vi "PID17.vi"() -> ()   [LabVIEW 2011]
uses:
  <vilib>/DAQmx/read.llb/DAQmx Read (Analog 1D DBL 1Chan NSamp).vi
  <vilib>/DAQmx/write.llb/DAQmx Write (Analog DBL 1Chan 1Samp).vi
  <vilib>/DAQmx/create/channels.llb/DAQmx Create Channel (AI-Voltage-Basic).vi
  <vilib>/DAQmx/configure/timing.llb/DAQmx Timing (Sample Clock).vi
  <vilib>/DAQmx/create/channels.llb/DAQmx Create Channel (AO-Voltage-Basic).vi
  <vilib>/DAQmx/miscellaneous.llb/DAQmx Fill In Error Info.vi
  <vilib>/express/express arith-compare/Formula/XNode/ExpressFormulaBlockNode.xnode
  <vilib>/Analysis/NI_AALBase.lvlib
  Program Files (x86)/National Instruments/LabVIEW 2011/resource/objmgr/daqmx.rc
panel:
  in  "error in":cluster{"status":bool}
  in  "?":T1(tab)
  out "Time":dbl
  out "Thermistor Back":dbl
  out "Thermistor Block":dbl
  out "Vial Ramp rate":dbl format="%#_3g"
  in  "stop":bool
  out "XY Graph":cluster{"Y":dbl[], "Y":dbl[]}[](graph)
  out "Setpoint":dbl
  in  "Zero":dbl=-0.6
  in  "Pole":dbl=-10000000000000.0
  in  "PID Heating":T2={"proportional gain (Kc)"=25.0, "integral time (Ti, s)"=6.0, "derivative time (Td, s)"=0.0} {"derivative time (Td, s)" format="%.3f"; "integral time (Ti, s)" format="%.3f"; "proportional gain (Kc)" format="%.3f"}
  out "Set Pt RampRate":dbl
  out "Error":dbl
  in  "PID Cooling":T2={"proportional gain (Kc)"=25.0, "integral time (Ti, s)"=6.0, "derivative time (Td, s)"=0.0} {"derivative time (Td, s)" format="%.3f"; "integral time (Ti, s)" format="%.3f"; "proportional gain (Kc)" format="%.3f"}
  out "Controller output":cluster{"Time Out":dbl[], dbl[]}(graph)
  out "Power Circuit":cluster{"Time Out":dbl[], dbl[]}(graph)
  out "Voltage":dbl
  out "Ave RR Up":dbl
  out "Ave RR Down":dbl
  in  "A 9":dbl=54.0
  in  "T 15":dbl=5.0
  in  "T 14":dbl=5.0
  in  "A 8":dbl=90.0
  in  "A 7":dbl=96.5
  in  "A 6":dbl=99.0
  in  "A 5":dbl=75.0
  in  "A 4":dbl=69.5
  in  "A 3":dbl=69.0
  in  "A 2":dbl=60.0
  in  "A 1":dbl=57.5
  in  "Aa 6":dbl=54.0
  in  "Aa 5":dbl=85.0
  in  "Aa 4":dbl=96.5
  in  "Aa 3":dbl=99.0
  in  "Aa 2":dbl=80.0
  in  "Aa 1":dbl=51.5
  in  "T 13":dbl=5.0
  in  "T 12":dbl=5.0
  in  "T 11":dbl=20.0
  in  "T 10":dbl=5.0
  in  "T 9":dbl=5.0
  in  "T 8":dbl=5.0
  in  "T 7":dbl=5.0
  in  "T 6":dbl=20.0
  in  "T 5":dbl=5.0
  in  "T 4":dbl=5.0
  in  "T 3":dbl=20.0
  in  "T 2":dbl=5.0
  in  "T 1":dbl=30.0
  in  "Ta 10":dbl=5.0
  in  "Ta 9":dbl=15.0
  in  "Ta 8":dbl=13.0
  in  "Ta 7":dbl=2.0
  in  "Ta 6":dbl=25.0
  in  "Ta 5":dbl=5.0
  in  "Ta 4":dbl=10.0
  in  "Ta 3":dbl=10.0
  in  "Ta 2":dbl=2.0
  in  "Ta 1":dbl=30.0
  in  "Graph Range":dbl=150.0
  out "Rate":dbl
  in  "Period(ms)":dbl=20.0
  out "time":dbl
  # "PID"
  # "Lead-Lag Compensator"
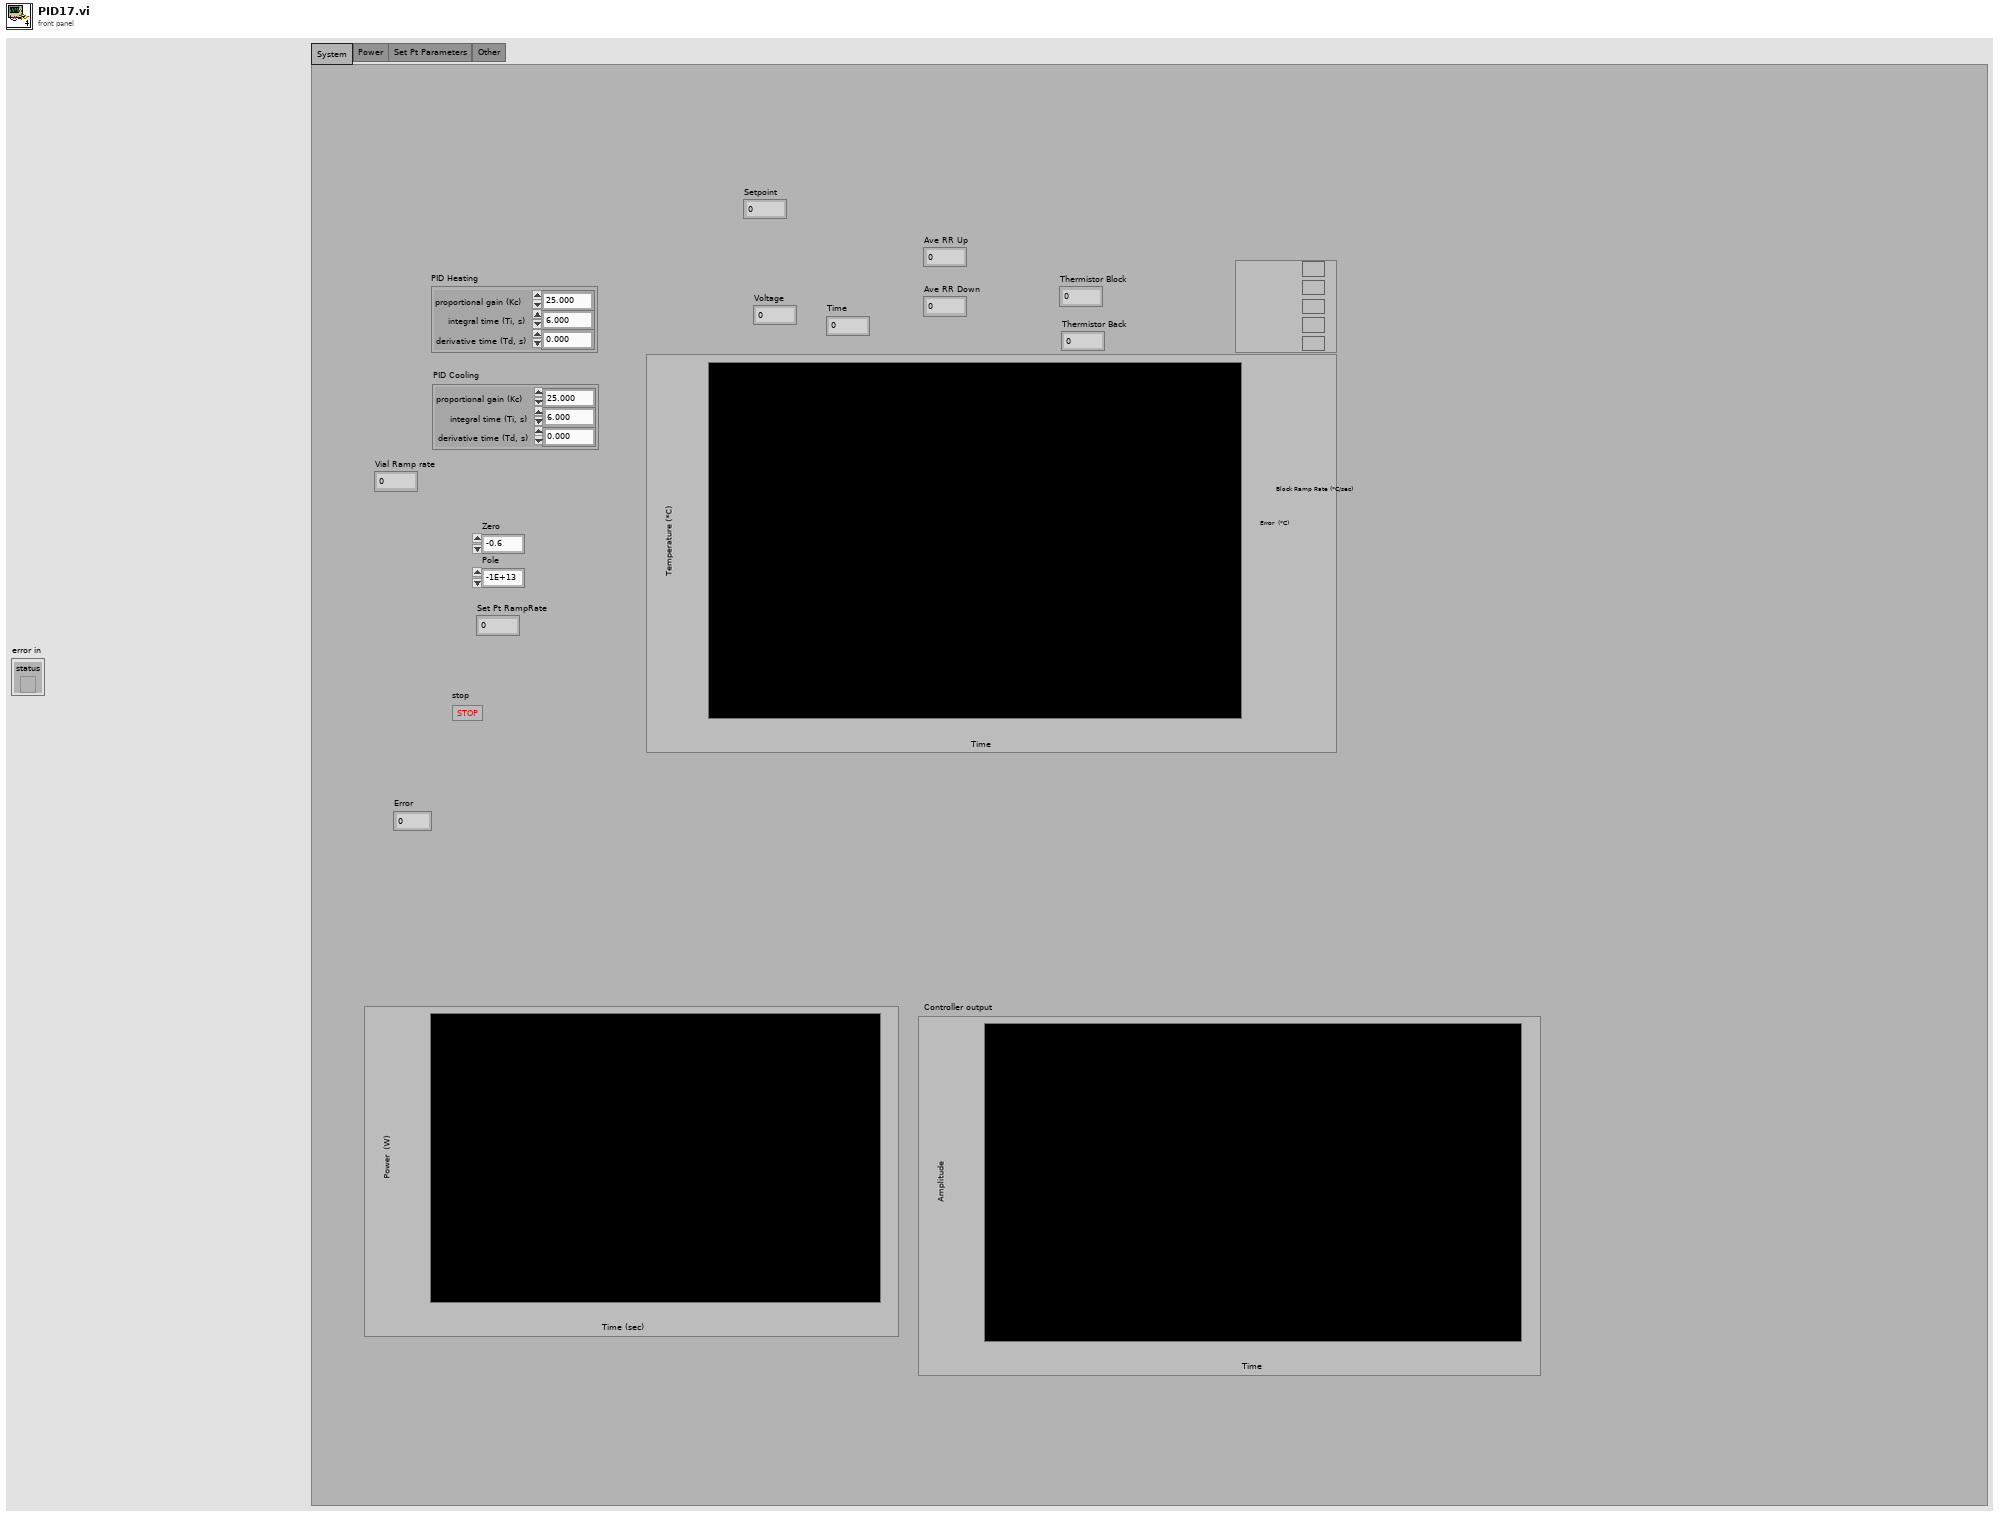
[diagram p1: front panel]
types:
  T1 = enum32{"System", "Power", "Set Pt Parameters", "Other"}
  T2 = cluster{"proportional gain (Kc)":dbl, "integral time (Ti, s)":dbl, "derivative time (Td, s)":dbl}
  T3 = enum16{"open", "replace", "create", "open or create", "replace or create", "replace or create with confirmation"}
  T4 = cluster{"x":dbl, "T1":dbl, "T2":dbl, "T3":dbl, "T4":dbl, "Te1":dbl, "Te2":dbl, "Te3":dbl, "Te4":dbl}
  T5 = cluster{"Ta 1":dbl, "Ta 2":dbl, "Ta 3":dbl, "Ta 4":dbl, "Ta 5":dbl, "Ta 6":dbl, "Ta 7":dbl, "Ta 8":dbl, "Ta 9":dbl, "Ta 10":dbl}
  T6 = cluster{"T 1":dbl, "T 2":dbl, "T 3":dbl, "T 4":dbl, "T 5":dbl, "T 6":dbl, "T 7":dbl, "T 8":dbl, "T 9":dbl, "T 10":dbl, "T 11":dbl, "T 12":dbl, "T 13":dbl, "T 14":dbl, "T 15":dbl}
  T7 = cluster{"Aa 1":dbl, "Aa 2":dbl, "Aa 3":dbl, "Aa 4":dbl, "Aa 5":dbl, "Aa 6":dbl, "A 1":dbl, "A 2":dbl, "A 3":dbl, "A 4":dbl, "A 5":dbl, "A 6":dbl, "A 7":dbl, "A 8":dbl, "A 9":dbl}
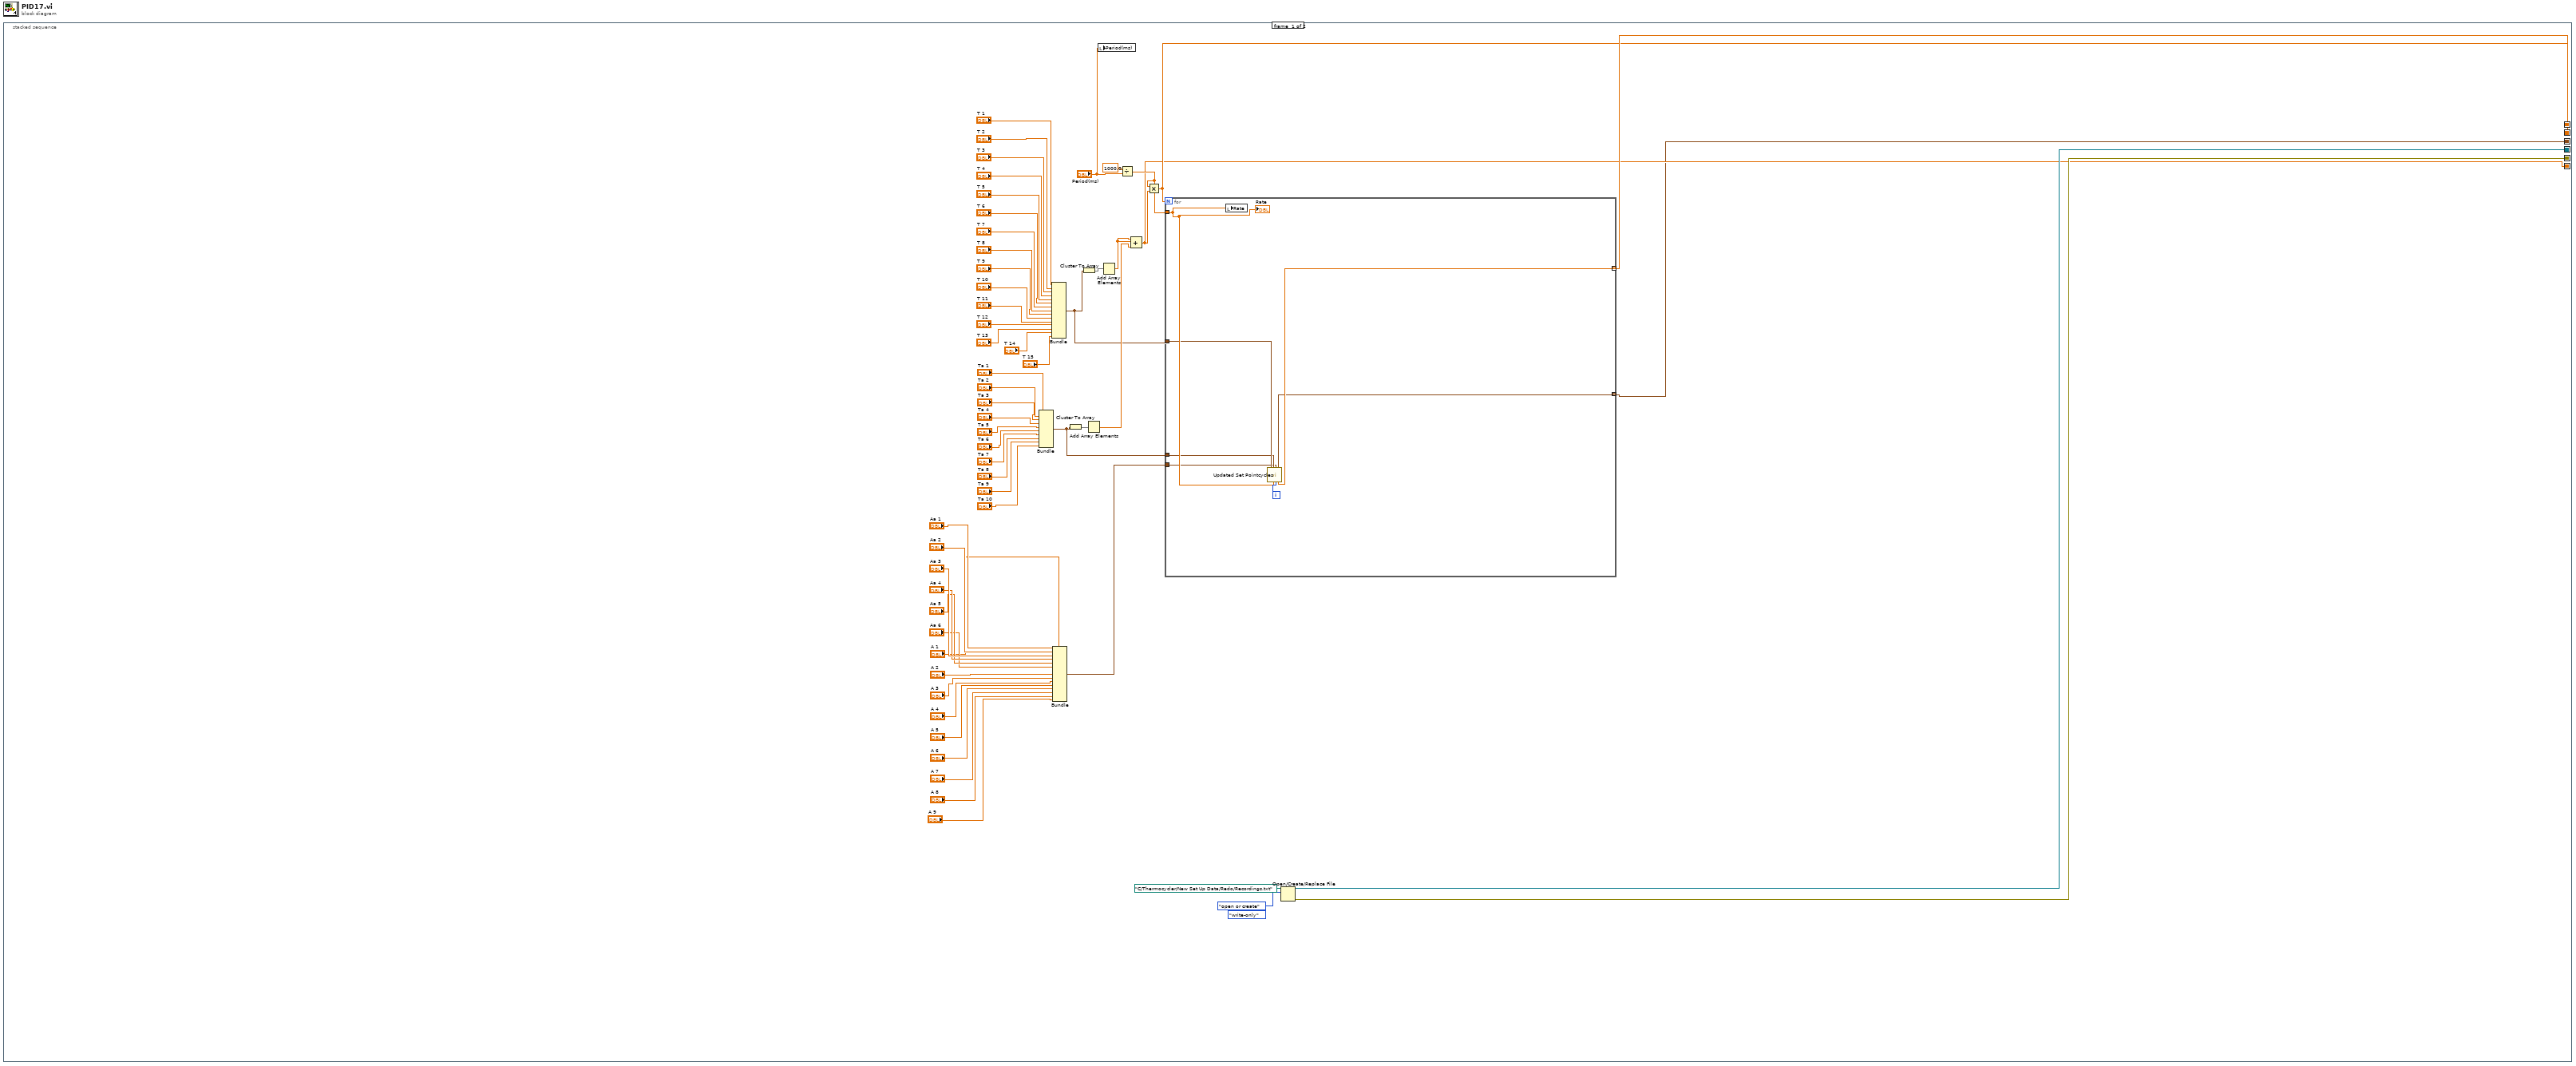
[diagram p0: block diagram]
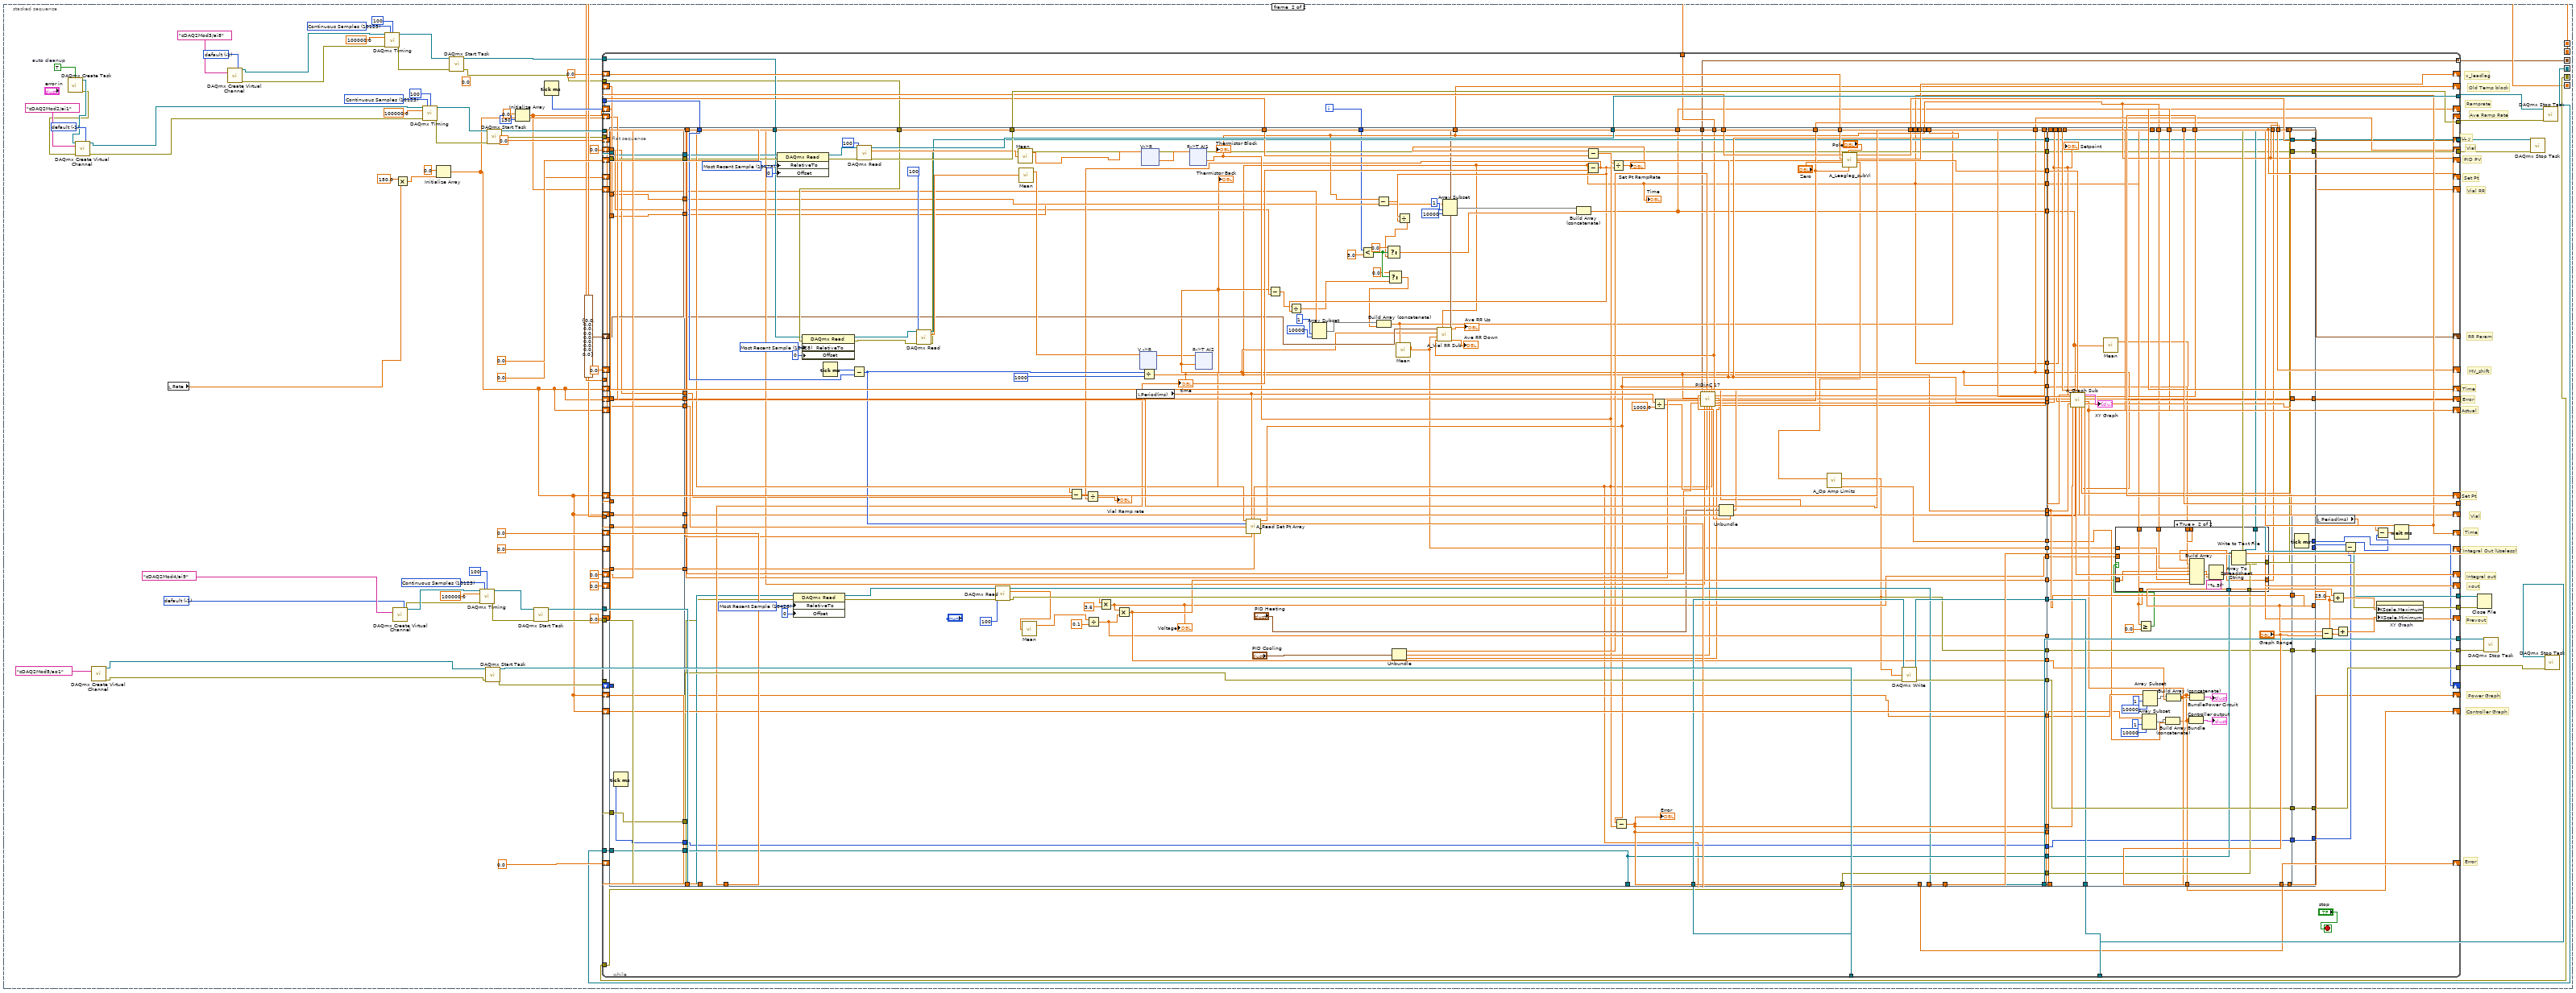
[diagram p2: hidden frame]
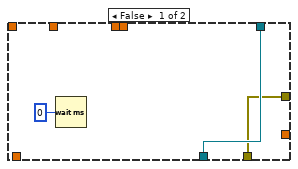
[diagram p3: hidden frame]
diagram:
  n1 = stacked-sequence {
    seq-local: [w57 _] -> [_ w132]
    seq-local: [w54 _] -> [_ w130]
    seq-local: [w4 _] -> [_ w66]
    seq-local: [w52 _] -> [_ w120]
    seq-local: [w51 _] -> [_ w119]
    seq-local: [w49 _] -> [_ w87]
    frame #0 {
      (unwired) enum16{"read/write", "read-only", "write-only"}."write-only" ("access (0:read/write)")
      n2 = Bundle("Ta 1"="Ta 1", "Ta 2"="Ta 2", "Ta 3"="Ta 3", "Ta 4"="Ta 4", "Ta 5"="Ta 5", "Ta 6"="Ta 6", "Ta 7"="Ta 7", "Ta 8"="Ta 8", "Ta 9"="Ta 9", "Ta 10"="Ta 10") -> (w20:T5)  [unwired: 1 in]
      n3 = Bundle("T 1"="T 1", "T 2"="T 2", "T 3"="T 3", "T 4"="T 4", "T 5"="T 5", "T 6"="T 6", "T 7"="T 7", "T 8"="T 8", "T 9"="T 9", "T 10"="T 10", "T 11"="T 11", "T 12"="T 12", "T 13"="T 13", "T 14"="T 14", "T 15"="T 15") -> (w21:T6)  [unwired: 1 in]
      n4 = Bundle("Aa 1"="Aa 1", "Aa 2"="Aa 2", "Aa 3"="Aa 3", "Aa 4"="Aa 4", "Aa 5"="Aa 5", "Aa 6"="Aa 6", "A 1"="A 1", "A 2"="A 2", "A 3"="A 3", "A 4"="A 4", "A 5"="A 5", "A 6"="A 6", "A 7"="A 7", "A 8"="A 8", "A 9"="A 9") -> (w5:T7)  [unwired: 1 in]
      n5 = Cluster To Array(cluster=w20) -> (array=w23:dbl[])
      n6 = Cluster To Array(cluster=w21) -> (array=w35:dbl[])
      n7 = Add Array Elements(numeric array=w23) -> (sum=w22:dbl)
      n8 = local write "Period(ms)"("Period(ms)") -> ()
      n9 = Add Array Elements(numeric array=w35) -> (sum=w34:dbl)
      n10 = Divide(x=1000.0, y="Period(ms)") -> (x/y=w55:dbl)
      n11 = Compound Arithmetic op=ADD(w34, w34, w22) -> (w49:dbl)
      n12 = Multiply(x=w55, y=w49) -> (x*y=w54:dbl)
      n13 = for {
        N: w54 -> [_]
        tunnel: w55 -> [w63]
        tunnel: [w65] -> w57 mode=indexing
        tunnel: w21 -> [w62]
        tunnel: w20 -> [w61]
        tunnel: w5 -> [w60]
        tunnel: [w59] -> w4 mode=indexing
        i -> [w64]
        n14 = local write "Rate"(w63) -> ()
        n15 = call "Updated Set Pointcycles.vi"("Time2"=w62, "Time1"=w61, "rate"=w63, "Amp"=w60, "i"=w64) -> ("Gain times"=w59:cluster{dbl, dbl, dbl, dbl, dbl, dbl}, "y"=w65:dbl)  [unwired: 13 in]
        "Rate" <- w63
      }
      n16 = Open/Create/Replace File(file path (use dialog)=path "C:/Thermocycler/New Set Up Data/Redo/Recordings.txt", operation (0:open)=T3."open or create") -> (refnum out=w52:refnum<file>, error out=w51:errorcluster)  [unwired: 2 in, 3 out]
    }
    frame #1 {
      w81 = -1 items=["default"=-1, "RSE"=10083, "NRSE"=10078, "Differential"=10106, "Pseudodifferential"=12529] ("input terminal configuration")
      (unwired) 0.0 ("y")
      w84 = 10123 items=["Finite Samples"=10178, "Continuous Samples"=10123, "Hardware Timed Single Point"=12522] ("sample mode")
      w103 = TRUE  # auto cleanup
      w105 = -1 items=["default"=-1, "RSE"=10083, "NRSE"=10078, "Differential"=10106, "Pseudodifferential"=12529] ("input terminal configuration")
      w112 = 10123 items=["Finite Samples"=10178, "Continuous Samples"=10123, "Hardware Timed Single Point"=12522] ("sample mode")
      w115 = -1 items=["default"=-1, "RSE"=10083, "NRSE"=10078, "Differential"=10106, "Pseudodifferential"=12529] ("input terminal configuration")
      w141 = 10123 items=["Finite Samples"=10178, "Continuous Samples"=10123, "Hardware Timed Single Point"=12522] ("sample mode")
      # "Vial RR"
      # "Vial"
      # "RR Param"
      # "Ave Ramp Rate"
      # "Ramprate"
      # "Old Temp block"
      # "Controller Graph"
      # "Power Graph"
      # "MV_shift"
      # "Prevout"
      # "xout"
      # "Integral out"
      # "Vial"
      # "Time"
      # "Integral Out (Useless)"
      # "Error"
      # "PID PV"
      # "Set Pt"
      # "x_leadlag"
      # "Set Pt"
      # "Actual"
      # "Error"
      # "Time"
      # "LL y"
      n17 = call <vilib>:"DAQmx Create Task.vi"("auto cleanup"=w103) -> ("task out"=w102:refnum<k21>, "error out"=w101:errorcluster)  [unwired: 13 in]
      n18 = call-poly <vilib>:"DAQmx Create Virtual Channel.vi"("task in"=w102, "input terminal configuration"=w105, "physical channels"=tag "cDAQ2Mod2/ai1", "error in"=w101) -> ("task out"=w86:refnum<k21>, "error out"=w85:errorcluster)  [unwired: 10 in]
      n19 = call-poly <vilib>:"DAQmx Create Virtual Channel.vi"("physical channels"=tag "cDAQ2Mod5/ao1") -> ("task out"=w95:refnum<k21>, "error out"=w94:errorcluster)  [unwired: 13 in]
      n20 = local read "Rate"() -> (w125:dbl)
      n21 = call-poly <vilib>:"DAQmx Create Virtual Channel.vi"("input terminal configuration"=w81, "physical channels"=tag "cDAQ2Mod3/ai8") -> ("task out"=w77:refnum<k21>, "error out"=w76:errorcluster)  [unwired: 12 in]
      n22 = call-poly <vilib>:"DAQmx Timing.vi"("task/channels in"=w77, "sample mode"=w84, "samples per channel"=100, "rate"=100000.0, "error in"=w76) -> ("task out"=w79:refnum<k21>, "error out"=w78:errorcluster)  [unwired: 9 in]
      n23 = call-poly <vilib>:"DAQmx Create Virtual Channel.vi"("input terminal configuration"=w115, "physical channels"=tag "cDAQ2Mod4/ai9") -> ("task out"=w114:refnum<k21>, "error out"=w113:errorcluster)  [unwired: 12 in]
      n24 = Multiply(x=150.0, y=w125) -> (x*y=w124:dbl)
      n25 = call-poly <vilib>:"DAQmx Timing.vi"("task/channels in"=w86, "sample mode"=w141, "samples per channel"=100, "rate"=100000.0, "error in"=w85) -> ("task out"=w99:refnum<k21>, "error out"=w98:errorcluster)  [unwired: 9 in]
      n26 = Initialize Array(0.0 ("element"), w124) -> (w69:dbl[])
      n27 = call <vilib>:"DAQmx Start Task.vi"("task/channels in"=w79, "error in"=w78) -> ("task out"=w75:refnum<k21>, "error out"=w74:errorcluster)  [unwired: 12 in]
      n28 = call-poly <vilib>:"DAQmx Timing.vi"("task/channels in"=w114, "sample mode"=w112, "samples per channel"=100, "rate"=100000.0, "error in"=w113) -> ("task out"=w97:refnum<k21>, "error out"=w96:errorcluster)  [unwired: 9 in]
      n29 = call <vilib>:"DAQmx Start Task.vi"("task/channels in"=w95, "error in"=w94) -> ("task out"=w131:refnum<k21>, "error out"=w137:errorcluster)  [unwired: 12 in]
      n30 = call <vilib>:"DAQmx Start Task.vi"("task/channels in"=w99, "error in"=w98) -> ("task out"=w139:refnum<k21>, "error out"=w100:errorcluster)  [unwired: 12 in]
      n31 = Initialize Array(0.0 ("element"), 150 ("dimension size")) -> (w68:dbl[])
      n32 = call <vilib>:"DAQmx Start Task.vi"("task/channels in"=w97, "error in"=w96) -> ("task out"=w109:refnum<k21>, "error out"=w108:errorcluster)  [unwired: 12 in]
      n33 = Tick Count (ms)() -> (millisecond timer value=w144:u32)
      n34 = while {
        tunnel: w144 -> [w280]
        shift-right: [w193] -> _
        shift-left: 0.0 ("data") -> [w258]
        shift-right: [w225] -> _
        shift-left: 0.0 -> [w277]
        tunnel: w100 -> [w275]
        tunnel: w139 -> [w274]
        tunnel: w137 -> [w271]
        tunnel: [w269] -> w136
        tunnel: [w266] -> w135
        tunnel: [w265] -> w134
        tunnel: [w264] -> w133
        tunnel: w132 -> [w263]
        tunnel: w131 -> [w261]
        tunnel: w130 -> [w259]
        shift-right: [w224] -> _
        shift-left: 0.0 ("Setpoint") -> [w233]
        shift-right: [w248] -> _
        shift-left: 0.0 ("Integral") -> [w255]
        tunnel: [w254] -> _
        shift-right: [w253] -> _
        shift-left: 0.0 -> [w252]
        shift-right: [w226] -> _
        shift-left: 0.0 ("y") -> [w250]
        shift-right: [w230] -> _
        shift-left: w69 -> [w246]
        shift-right: [w229] -> _
        shift-left: w69 -> [w243]
        shift-right: [w227] -> _
        shift-left: w69 -> [w242]
        shift-right: [w228] -> _
        shift-left: w69 -> [w247]
        shift-right: [w236] -> _
        shift-left: 0.0 ("LL x out") -> [w235]
        tunnel: w120 -> [w223]
        tunnel: w119 -> [w220]
        tunnel: [w218] -> w118
        tunnel: [w217] -> w117
        tunnel: w109 -> [w216]
        tunnel: w108 -> [w215]
        tunnel: [w214] -> w107
        tunnel: [w213] -> w106
        shift-right: [w208] -> _
        shift-left: w69 -> [w207]
        shift-right: [w203] -> _
        shift-left: 0.0 ("Integral out") -> [w199]
        shift-right: [w202] -> _
        shift-left: 0.0 ("x out") -> [w198]
        shift-right: [w201] -> _
        shift-left: 0.0 ("prev out") -> [w200]
        shift-right: [w197] -> _
        shift-left: 0.0 ("MV") -> [w196]
        shift-right: [w195] -> _
        shift-left: 0.0 ("Result") -> [w151]
        shift-right: [w187] -> _
        shift-left: _ -> [w186]
        shift-right: [w180] -> _
        shift-left: w69 -> [w182]
        shift-right: [w178] -> _
        shift-left: w69 -> [w179]
        tunnel: w87 -> [w175]
        tunnel: w75 -> [w174]
        tunnel: w74 -> [w167]
        tunnel: [w171] -> w73
        tunnel: [w168] -> w72
        shift-right: [w166] -> _
        shift-left: _ -> [w165]
        shift-right: [w163] -> _
        shift-left: w68 -> [w162]
        shift-right: [w159] -> _
        shift-left: w69 -> [w157]
        shift-right: [w153] -> _
        shift-left: T4 {"x"=0.0, "T1"=0.0, "T2"=0.0, "T3"=0.0, "T4"=0.0, "Te1"=0.0, "Te2"=0.0, "Te3"=0.0, "Te4"=0.0} ("Param out") -> [w152]
        shift-right: [w150] -> _
        shift-left: w68 -> [w149]
        tunnel: w66 -> [w145] mode=indexing
        i -> [w147]
        stop <- "stop" stop-if-true
        w241 = 25.0 ("y")
        n35 = flat-sequence {
          tunnel: [w293] -> w276
          tunnel: w275 -> [w293]
          tunnel: w274 -> [w290]
          tunnel: [w290] -> w273
          tunnel: [w292] -> w272
          tunnel: w271 -> [w292]
          tunnel: w263 -> [w291]
          tunnel: [w291] -> w262
          tunnel: [w289] -> w260
          tunnel: w259 -> [w289]
          tunnel: [w288] -> w256
          tunnel: w255 -> [w288]
          tunnel: w223 -> [w287]
          tunnel: [w287] -> w222
          tunnel: w207 -> [w286]
          tunnel: [w286] -> w206
          tunnel: [w285] -> w194
          tunnel: w151 -> [w285]
          tunnel: [w284] -> w191
          tunnel: w186 -> [_]
          tunnel: w165 -> [w283]
          tunnel: [w283] -> w164
          tunnel: w162 -> [w282]
          tunnel: [w282] -> w161
          tunnel: w157 -> [w281]
          tunnel: [w281] -> w156
          tunnel: w280 -> [w414]
          tunnel: [w348] -> w279
          tunnel: [w296] -> w278
          tunnel: [w296] -> w225
          tunnel: w277 -> [w391]
          tunnel: w276 -> [w386]
          tunnel: w273 -> [w412]
          tunnel: w272 -> [w411]
          tunnel: [w410] -> w270
          tunnel: [w409] -> w267
          tunnel: [w408] -> w265
          tunnel: [w407] -> w264
          tunnel: w262 -> [w406]
          tunnel: w261 -> [w405]
          tunnel: w260 -> [w404]
          tunnel: [w331] -> w193
          tunnel: w258 -> [w403]
          tunnel: [w331] -> w257
          tunnel: w233 -> [w395]
          tunnel: [w348] -> w224
          tunnel: [w402] -> w248
          tunnel: w256 -> [w401]
          tunnel: [w331] -> _
          tunnel: [w394] -> w253
          tunnel: w252 -> [_]
          tunnel: [w394] -> w251
          tunnel: [w397] -> w226
          tunnel: w250 -> [w398]
          tunnel: [w392] -> w236
          tunnel: [w296] -> w245
          tunnel: [w394] -> w244
          tunnel: w235 -> [w393]
          tunnel: w222 -> [w390]
          tunnel: [w390] -> _
          tunnel: [w390] -> w221
          tunnel: w220 -> [w389]
          tunnel: [w389] -> w219
          tunnel: w216 -> [w388]
          tunnel: w215 -> [w385]
          tunnel: [w381] -> w214
          tunnel: [w380] -> w212
          tunnel: [w377] -> w210
          tunnel: [w377] -> w209
          tunnel: w206 -> [w376]
          tunnel: [w376] -> w205
          tunnel: [w308] -> w204
          tunnel: [w370] -> w203
          tunnel: [w369] -> w202
          tunnel: [w368] -> w201
          tunnel: w200 -> [w367]
          tunnel: w199 -> [w366]
          tunnel: w198 -> [w365]
          tunnel: [w364] -> w197
          tunnel: w196 -> [_]
          tunnel: [w308] -> w195
          tunnel: w194 -> [w363]
          tunnel: [w308] -> w192
          tunnel: w191 -> [w358]
          tunnel: [w358] -> w190
          tunnel: w182 -> [w357]
          tunnel: [w357] -> w181
          tunnel: [w355] -> w177
          tunnel: [w354] -> w176
          tunnel: w175 -> [w316]
          tunnel: w174 -> [w335]
          tunnel: [w340] -> w173
          tunnel: [w339] -> w170
          tunnel: w167 -> [w336]
          tunnel: [w331] -> w166
          tunnel: w164 -> [w330]
          tunnel: [w326] -> w163
          tunnel: w161 -> [w327]
          tunnel: [w326] -> w160
          tunnel: w156 -> [w325]
          tunnel: [w325] -> w155
          tunnel: [w322] -> w154
          tunnel: [w319] -> w153
          tunnel: w152 -> [w318]
          tunnel: w151 -> [w314]
          tunnel: [w310] -> w150
          tunnel: w149 -> [w309]
          tunnel: [w299] -> w148
          tunnel: w147 -> [w305]
          tunnel: [w296] -> w146
          tunnel: w145 -> [w295]
          tunnel: w279 -> [w496]
          tunnel: w278 -> [w486]
          tunnel: w270 -> [w509]
          tunnel: [w509] -> w268
          tunnel: w267 -> [w508]
          tunnel: [w508] -> w266
          tunnel: w257 -> [w498]
          tunnel: [w486] -> _
          tunnel: [w496] -> w254
          tunnel: w251 -> [_]
          tunnel: "Graph Range" -> [_]
          tunnel: [w506] -> w228
          tunnel: w247 -> [w505]
          tunnel: w246 -> [w504]
          tunnel: [w468] -> w230
          tunnel: w245 -> [w497]
          tunnel: w244 -> [w503]
          tunnel: w243 -> [w502]
          tunnel: [w501] -> w229
          tunnel: [w500] -> w227
          tunnel: w242 -> [w499]
          tunnel: [w497] -> w240
          tunnel: w225 -> [w493]
          tunnel: w224 -> [w492]
          tunnel: w193 -> [_]
          tunnel: w221 -> [w491]
          tunnel: w219 -> [w490]
          tunnel: [w489] -> w218
          tunnel: [w488] -> w217
          tunnel: w212 -> [w487]
          tunnel: [w487] -> w211
          tunnel: w210 -> [w473]
          tunnel: w209 -> [w485]
          tunnel: [w484] -> w208
          tunnel: w205 -> [w483]
          tunnel: w204 -> [w482]
          tunnel: w193 -> [w481]
          tunnel: w192 -> [w479]
          tunnel: w190 -> [w480]
          tunnel: [w480] -> w189
          tunnel: w181 -> [w472]
          tunnel: [w471] -> w180
          tunnel: w179 -> [w465]
          tunnel: [w464] -> w178
          tunnel: w177 -> [w463]
          tunnel: w176 -> [_]
          tunnel: w173 -> [w462]
          tunnel: [w462] -> w172
          tunnel: w170 -> [w461]
          tunnel: [w461] -> w169
          tunnel: w160 -> [w458]
          tunnel: [w460] -> w158
          tunnel: w155 -> [w459]
          tunnel: w154 -> [w467]
          tunnel: w148 -> [w456]
          tunnel: w146 -> [w455]
          tunnel: [w530] -> w232
          tunnel: [w534] -> w269
          tunnel: w268 -> [w534]
          tunnel: w240 -> [w533]
          tunnel: [w533] -> w238
          tunnel: [w532] -> w213
          tunnel: w211 -> [w532]
          tunnel: w189 -> [w531]
          tunnel: [w531] -> w188
          tunnel: [w530] -> w187
          tunnel: w172 -> [w529]
          tunnel: [w529] -> w171
          tunnel: w169 -> [w528]
          tunnel: [w528] -> w168
          tunnel: [w527] -> w159
          tunnel: w158 -> [w527]
          frame #0 {
            n36 = Tick Count (ms)() -> (millisecond timer value=w284:u32)
          }
          frame #1 {
            w337 = 10428 items=["First Sample"=10424, "Current Read Position"=10425, "Reference Trigger"=10426, "First Pretrigger Sample"=10427, "Most Recent Sample"=10428] ("RelativeTo")
            w382 = 10428 items=["First Sample"=10424, "Current Read Position"=10425, "Reference Trigger"=10426, "First Pretrigger Sample"=10427, "Most Recent Sample"=10428] ("RelativeTo")
            w419 = 10428 items=["First Sample"=10424, "Current Read Position"=10425, "Reference Trigger"=10426, "First Pretrigger Sample"=10427, "Most Recent Sample"=10428] ("RelativeTo")
            n37 = property class="DAQmx Read"(reference=w412, error in=w386, "RelativeTo"=w419, "Offset"=0) -> (reference out=w417:refnum<k21>, error out=w416:errorcluster)
            n38 = property class="DAQmx Read"(reference=w388, error in=w385, "RelativeTo"=w382, "Offset"=0) -> (reference out=w387:refnum<k21>, error out=w384:errorcluster)
            n39 = property class="DAQmx Read"(reference=w335, error in=w336, "RelativeTo"=w337, "Offset"=0) -> (reference out=w334:refnum<k21>, error out=w333:errorcluster)
            n40 = Tick Count (ms)() -> (millisecond timer value=w420:u32)
            n41 = Subtract(x=w420, y=w414) -> (x-y=w396:u32)
            n42 = call-poly <vilib>:"DAQmx Read.vi"("task/channels in"=w417, "number of samples per channel"=100, "error in"=w416) -> ("task out"=w408:refnum<k21>, "data"=w343:dbl[], "error out"=w407:errorcluster)  [unwired: 10 in]
            n43 = call-poly <vilib>:"DAQmx Read.vi"("task/channels in"=w334, "number of samples per channel"=100, "error in"=w333) -> ("task out"=w340:refnum<k21>, "data"=w341:dbl[], "error out"=w339:errorcluster)  [unwired: 10 in]
            n44 = call-poly <vilib>:"DAQmx Read.vi"("task/channels in"=w387, "number of samples per channel"=100, "error in"=w384) -> ("task out"=w381:refnum<k21>, "data"=w345:dbl[], "error out"=w380:errorcluster)  [unwired: 10 in]
            n45 = call <vilib>:"Mean.vi"("X"=w343) -> ("mean"=w347:dbl)  [unwired: 1 out]
            n46 = call <vilib>:"Mean.vi"("X"=w341) -> ("mean"=w375:dbl)  [unwired: 1 out]
            n47 = call <vilib>:"Mean.vi"("X"=w345) -> ("mean"=w344:dbl)  [unwired: 1 out]
            n48 = Divide(x=w344, y=0.1) -> (x/y=w354:dbl)
            n49 = local read "Period(ms)"() -> (w361:dbl)
            n50 = xnode "V ->R"("V"=w375) -> ("Result"=w307:dbl)  [unwired: 1 in, 1 out]
            n51 = xnode "V->R"("V"=w347) -> ("Result"=w422:dbl)  [unwired: 1 in, 1 out]
            n52 = Divide(x=w396, y=1000) -> (x/y=w296:dbl)
            "time" <- w296
            "Time" <- w296
            n53 = xnode "R->T AI1"("R"=w422) -> ("Result"=w331:dbl)  [unwired: 1 in, 1 out]
            "Thermistor Block" <- w331
            n54 = xnode "R->T AI2"("R"=w307) -> ("Result"=w308:dbl)  [unwired: 1 in, 1 out]
            "Thermistor Back" <- w308
            n55 = Subtract(x=w308, y=w363) -> (x-y=w362:dbl)
            n56 = call "A_Read Set Pt Array.vi"("Previous y"=w403, "Period(ms)"=w361, "Result"=w331, "dt"=w396, "y array"=w406, "arraysize"=w404, "Integral in"=w401) -> ("Set Pt Out"=w348:dbl, "Integral out"=w402:dbl)  [unwired: 7 in]
            n57 = Subtract(x=w308, y=w314) -> (x-y=w313:dbl)
            n58 = Array Subset(array=w309, index=1, length=10000) -> (w315:dbl[])
            n59 = Less?(x=w305, y=5.0) -> (x < y?=w303:bool)
            n60 = Subtract(x=w331, y=w330) -> (x-y=w332:dbl)
            n61 = Unbundle("PID Cooling") -> ("proportional gain (Kc)"=w352:dbl, "integral time (Ti, s)"=w350:dbl, "derivative time (Td, s)"=w351:dbl)
            n62 = Array Subset(array=w327, index=1, length=10000) -> (w328:dbl[])
            n63 = Subtract(x=w348, y=w395) -> (x-y=w413:dbl)
            n64 = Subtract(x=w296, y=w391) -> (x-y=w317:dbl)
            n65 = Divide(x=w362, y=w317) -> (x/y=→"Vial Ramp rate":dbl)
            n66 = Divide(x=w313, y=w317) -> (x/y=w298:dbl)
            n67 = Select(t=0.0, s=w303, f=w298) -> (s? t:f=w297:dbl)
            n68 = Build Array (concatenate)(w315, w297) -> (w310:dbl[])
            n69 = call <vilib>:"Mean.vi"("X"=w310) -> ("mean"=w299:dbl)  [unwired: 1 out]
            n70 = Divide(x=w332, y=w317) -> (x/y=w301:dbl)
            n71 = Select(t=0.0, s=w303, f=w301) -> (s? t:f=w300:dbl)
            n72 = call "A_Vial RR Sub.vi"("t"=w296, "TotalTime"=w316, "Vial Slope"=w299, "Vial Temp"=w308, "Param in"=w318) -> ("Ave RR Down"=→"Ave RR Down":dbl, "Param out"=w319:T4, "Ave RR Up"=→"Ave RR Up":dbl)  [unwired: 4 in]
            n73 = Build Array (concatenate)(w328, w300) -> (w326:dbl[])
            n74 = Divide(x=w413, y=w317) -> (x/y=→"Set Pt RampRate":dbl)
            n75 = Subtract(x=w348, y=w331) -> (x-y=w394:dbl)
            "Error" <- w394
            n76 = Divide(x=w361, y=1000.0) -> (x/y=w360:dbl)
            n77 = Unbundle("PID Heating") -> ("proportional gain (Kc)"=w372:dbl, "integral time (Ti, s)"=w373:dbl, "derivative time (Td, s)"=w374:dbl)
            n78 = call "PIDinC 17.vi"("Gain Schedule"=w295, "D"=w374, "Time"=w296, "Integral in"=w366, "prev in"=w367, "I"=w373, "x in"=w365, "P2"=w352, "dt"=w360, "P"=w372, "I2"=w350, "Set Point"=w348, "PV"=w331, "Total Time"=w316, "D2"=w351) -> ("Integral out"=w370:dbl, "MV"=w364:dbl, "prev out"=w368:dbl, "x out"=w369:dbl)  [unwired: 1 in]
            n79 = call "A_Leaglag_subVi.vi"("LL x"=w364, "Pole"="Pole", "Zero"="Zero", "LL x_prev"=w393, "LL y_prev"=w398) -> ("y*inv_gain"=w323:dbl, "LL x out"=w392:dbl, "LL y"=w397:dbl)  [unwired: 4 in]
            n80 = call "A_Op Amp Limits.vi"("Lead Lag"=w323) -> ("Controller Output"=w322:dbl, "Write DAQmx"=w294:dbl)  [unwired: 9 in]
            n81 = Multiply(x=w294, y=3.6) -> (x*y=w355:dbl)
            "Voltage" <- w355
            n82 = Multiply(x=w355, y=w354) -> (x*y=w377:dbl)
            n83 = call-poly <vilib>:"DAQmx Write.vi"("task/channels in"=w405, "data"=w294, "error in"=w411) -> ("task out"=w409:refnum<k21>, "error out"=w410:errorcluster)  [unwired: 10 in, 1 out]
          }
          frame #2 {
            n84 = call "A_Graph Sub.vi"("Set Point Shift"=w505, "New Set Pt"=w496, "Ramp Rate Shift"=w459, "Time Shift"=w504, "New Time"=w497, "New Error"=w503, "New Ramp Rate"=w458, "Error Shift"=w502, "New Actual"=w498, "Actual Shift"=w499, "New Vial"=w482, "Vial Shift"=w483) -> ("Vial Out"=w484:dbl[], "Actual Out"=w500:dbl[], "Graph Out"=→"XY Graph":cluster{dbl[], dbl[]}[], "Set Pt Out"=w506:dbl[], "Ramp Rate Out"=w460:dbl[], "Time Out"=w468:dbl[], "Error Out"=w501:dbl[])  [unwired: 1 in]
            n85 = call <vilib>:"Mean.vi"("X"=w458) -> ("mean"=w457:dbl)  [unwired: 1 out]
            n86 = Greater Or Equal?(x=w493, y=0.0) -> (x >= y?=w494:bool)
            n87 = case shown="True" w494 {
              tunnel: w493 -> [_ _]
              tunnel: w492 -> [_ w516]
              tunnel: w491 -> [w511 w526]
              tunnel: w490 -> [w510 w525]
              tunnel: [w510 w524] -> w489
              tunnel: [w511 w523] -> w488
              tunnel: w485 -> [_ w519]
              tunnel: w481 -> [_ w518]
              tunnel: w479 -> [_ w517]
              tunnel: w463 -> [_ _]
              tunnel: w457 -> [_ w515]
              tunnel: w456 -> [_ w514]
              tunnel: w455 -> [_ w513]
              frame False {
                n88 = Wait (ms)(milliseconds to wait=u32 0) -> ()  [unwired: 1 out]
              }
              frame True {
                n89 = Build Array(w516, w517, w518, w519, w515, w514, w513) -> (w522:dbl[])
                n90 = Array To Spreadsheet String(array=w522, 3:"%.5f" ("format string")) -> (spreadsheet string=w520:string)  [unwired: 1 out]
                n91 = Write to Text File(file (use dialog)=w526, text=w520, error in=w525) -> (refnum out=w523:refnum<file>, error out=w524:errorcluster)  [unwired: 1 in, 1 out]
              }
            }
            n92 = Array Subset(array=w465, index=1, length=10000) -> (w466:dbl[])
            n93 = Array Subset(array=w472, index=1, length=10000) -> (w470:dbl[])
            n94 = Build Array (concatenate)(w466, w467) -> (w464:dbl[])
            n95 = Build Array (concatenate)(w470, w473) -> (w471:dbl[])
            n96 = Bundle("Time Out"=w468, w464) -> (→"Controller output":cluster{"Time Out":dbl[], dbl[]})  [unwired: 1 in]
            n97 = Bundle("Time Out"=w468, w471) -> (→"Power Circuit":cluster{"Time Out":dbl[], dbl[]})  [unwired: 1 in]
            "Setpoint" <- w496
          }
          frame #3 {
            n98 = Tick Count (ms)() -> (millisecond timer value=w530:u32)
          }
        }
        n99 = local read "Period(ms)"() -> (w185:dbl)
        n100 = Subtract(x=w238, y="Graph Range") -> (x-y=w249:dbl)
        n101 = Add(x=w238, y=w241) -> (x+y=w239:dbl)
        n102 = Add(x=w241, y=w249) -> (x+y=w237:dbl)
        n103 = Subtract(x=w232, y=w188) -> (x-y=w183:u32)
        n104 = Subtract(x=w185, y=w183) -> (x-y=w184:dbl)
        n105 = property on="XY Graph" class="XYGraph (strict)"("XScale.Maximum"=w239, "XScale.Minimum"=w237) -> ()  [unwired: 2 in, 2 out]
        n106 = Wait (ms)(milliseconds to wait=w184) -> ()  [unwired: 1 out]
      }
      n107 = Close File(refnum=w117, error in=w118) -> ()  [unwired: 2 out]
      n108 = call <vilib>:"DAQmx Stop Task.vi"("task/channels in"=w107, "error in"=w106) -> ()  [unwired: 12 in, 2 out]
      n109 = call <vilib>:"DAQmx Stop Task.vi"("task/channels in"=w73, "error in"=w72) -> ()  [unwired: 12 in, 2 out]
      n110 = call <vilib>:"DAQmx Stop Task.vi"("task/channels in"=w134, "error in"=w133) -> ()  [unwired: 12 in, 2 out]
      n111 = call <vilib>:"DAQmx Stop Task.vi"("task/channels in"=w135, "error in"=w136) -> ()  [unwired: 12 in, 2 out]
    }
  }
